vi "Test Format Into String Multiple.vi"() -> ()   [LabVIEW 2021]
doc: "VI for testing the results of custom VI which allows to format multiple input values into one string."
panel:
  out "Formated String":string
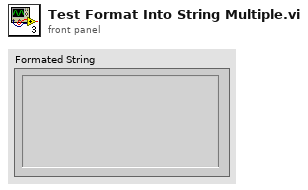
[diagram p1: front panel]
types:
  T1 = cluster{string, u16[], "element":u16, cluster{string, bool, i32[]}}
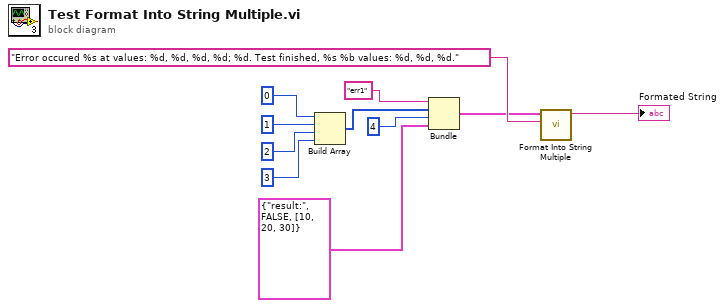
[diagram p0: block diagram]
diagram:
  n1 = Build Array(u16 0 ("element"), u16 1 ("element"), u16 2 ("element"), u16 3 ("element")) -> (w5:u16[])
  n2 = Bundle("err1", w5, "element"=u16 4, cluster{string, bool, i32[]} {"result:", FALSE, [10, 20, 30]}) -> (w1:T1)  [unwired: 1 in]
  n3 = call "Format Into String Multiple.vi"("Format String"="Error occured %s at values: %d, %d, %d, %d; %d. Test finished, %s %b values: %d, %d, %d.", "Input Values"=w1) -> ("Formated String"=→"Formated String":string)  [unwired: 8 in, 1 out]
